vi "Pre Launch Init.vi"(11 "uService Template in":refnum<class "Kasli Wrapper 2.0.lvclass">) -> (0 "error out":errorcluster, 3 "uService Template out":refnum<class "Kasli Wrapper 2.0.lvclass">)   [LabVIEW 2020, in "TALOS.lvlib" / "Kasli Wrapper 2.0.lvlib" / "Kasli Wrapper 2.0.lvclass"]
doc: "(<B>Filename</B>: Actor Framework.lvlib:Actor.lvclass:Pre Launch Init.vi)\n\nDefines behavior that occurs after the Launch Nested Actor method is invoked but before the actor's Actor Core method begins running.\n\nBy default, this method does nothing. A descendant class may override it to define behavior."
uses:
  Kasli Wrapper 2.0.lvclass
  Kasli Wrapper 2.0.lvclass/Kasli Wrapper 2.0.ctl
  Father of all uServices/Father of all uServices/Father of all uServices.lvclass
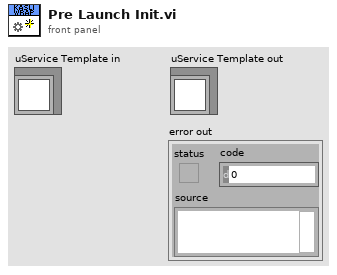
[diagram p1: front panel]
types:
  T1 = cluster{"stdout event":refnum<user-event>, "stderr event":refnum<user-event>, "process_exit event":refnum<user-event>}
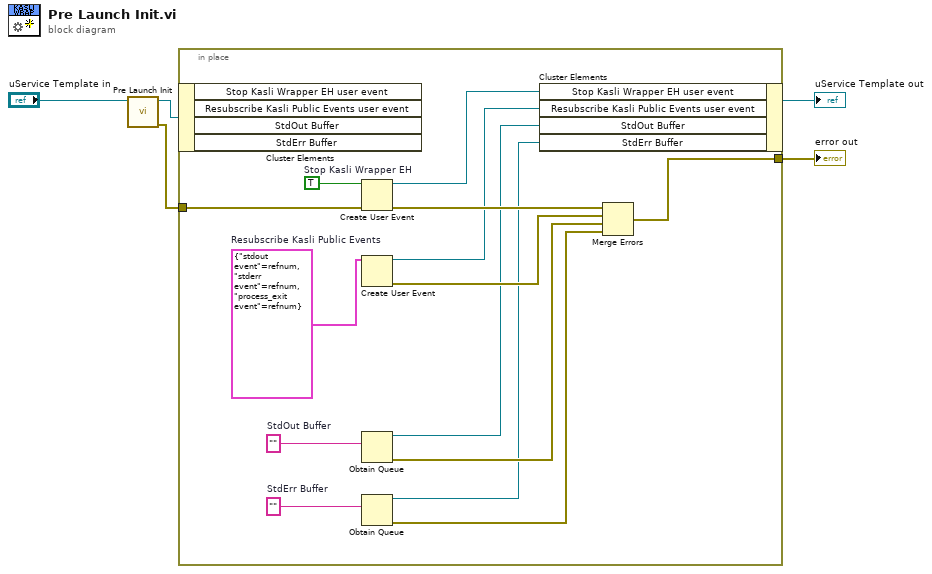
[diagram p0: block diagram]
diagram:
  n1 = call-parent "Pre Launch Init.vi"("uService Template in"="uService Template in") -> ("error out"=w4:errorcluster, "uService Template out"=w3:refnum<class "Kasli Wrapper 2.0.lvclass">)  [unwired: 9 in]
  n2 = in-place {
    in-place-border: w4 -> [w18]
    in-place-border: [w15] -> w2
    w10 = ""  # StdErr Buffer
    w11 = ""  # StdOut Buffer
    w13 = T1 {"stdout event"=refnum, "stderr event"=refnum, "process_exit event"=refnum}  # Resubscribe Kasli Public Events
    w19 = TRUE  # Stop Kasli Wrapper EH
    n3 = in-place-cluster #1(w3) -> ()  [unwired: 4 out]
    n4 = Create User Event(user event datatype=w19, error in=w18) -> (user event=w17:refnum<user-event>, error out=w16:errorcluster)
    n5 = Create User Event(user event datatype=w13) -> (user event=w12:refnum<user-event>, error out=w14:errorcluster)  [unwired: 1 in]
    n6 = Obtain Queue(element data type=w11) -> (queue out=w8:refnum<queue>, error out=w9:errorcluster)  [unwired: 4 in, 1 out]
    n7 = Obtain Queue(element data type=w10) -> (queue out=w7:refnum<queue>, error out=w6:errorcluster)  [unwired: 4 in, 1 out]
    n8 = in-place-cluster #1("Stop Kasli Wrapper EH user event"=w17, "Resubscribe Kasli Public Events user event"=w12, "StdOut Buffer"=w8, "StdErr Buffer"=w7) -> (→"uService Template out":refnum<class "Kasli Wrapper 2.0.lvclass">)
    n9 = Merge Errors(w16, w14, w9, w6) -> (w15:errorcluster)
  }
  "error out" <- w2
